vi "Initialize Core.vi"(8 "Error In":errorcluster, 11 "CS++MessageLogger in":refnum<class "CS++MessageLogger.lvclass">) -> (0 "Error Out":errorcluster, 3 "CS++MessageLogger out":refnum<class "CS++MessageLogger.lvclass">)   [LabVIEW 2014, in "CS++BaseClasses.lvlib" / "CS++MessageLogger.lvclass"]
doc: "Initialize the message logger."
uses:
  CS++MessageLogger.lvclass
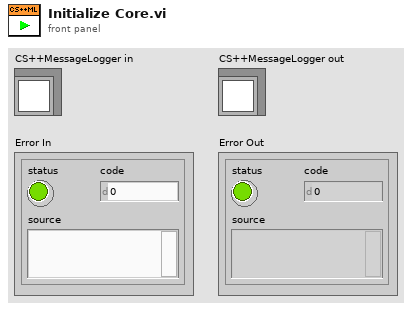
[diagram p1: front panel]
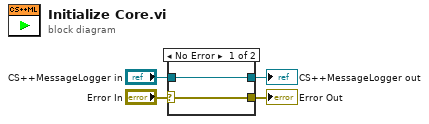
[diagram p0: block diagram]
diagram:
  n1 = case shown="No Error" "Error In" {
    selector: "Error In" -> [w5 w8]
    tunnel: [w5 w8] -> w3
    tunnel: [w6 w7] -> w1
    tunnel: "CS++MessageLogger in" -> [w6 w7]
    frame No Error {
    }
    frame Error {
    }
  }
  "Error Out" <- w3
  "CS++MessageLogger out" <- w1
